vi "02Manejo_panel 568.vi"(0 "Config Equipos":T2(array[cluster]) {"Ref PD" max=10000 step=1; "Med Princ" items=["1", "2", "3", "4", "5", "6", "7", "8", "9", "10", "11", "12", "13", "14", "15", "16", "17", "18", "19", "20", "21", "22", "23", "24", "25", "26", "27", "28", "29", "30", "31", "32"]}, 2 "Med EQ 568":T1, 3 "Nº equipo":i32, 4 "Paneles in":T4(array[cluster]) {"Nº" min=1.0 max=60.0 step=1.0 format="%#2.1f"; "Ultima recepción" format="%<%d/%m - %X>T"; "Med\nPpal" format="%_4g"}) -> (5 "Paneles out":T3(array[cluster]) {"Numeric" min=1.0 max=60.0 step=1.0 format="%#2.1f"; "Ultima recepción" format="%<%d/%m - %X>T"; "Med\nPpal" format="%_4g"})   [LabVIEW 2010]
panel:
  in  "Flags recep":bool[](array[boolean])
  out "T. error":timestamp[](array[timestamp])
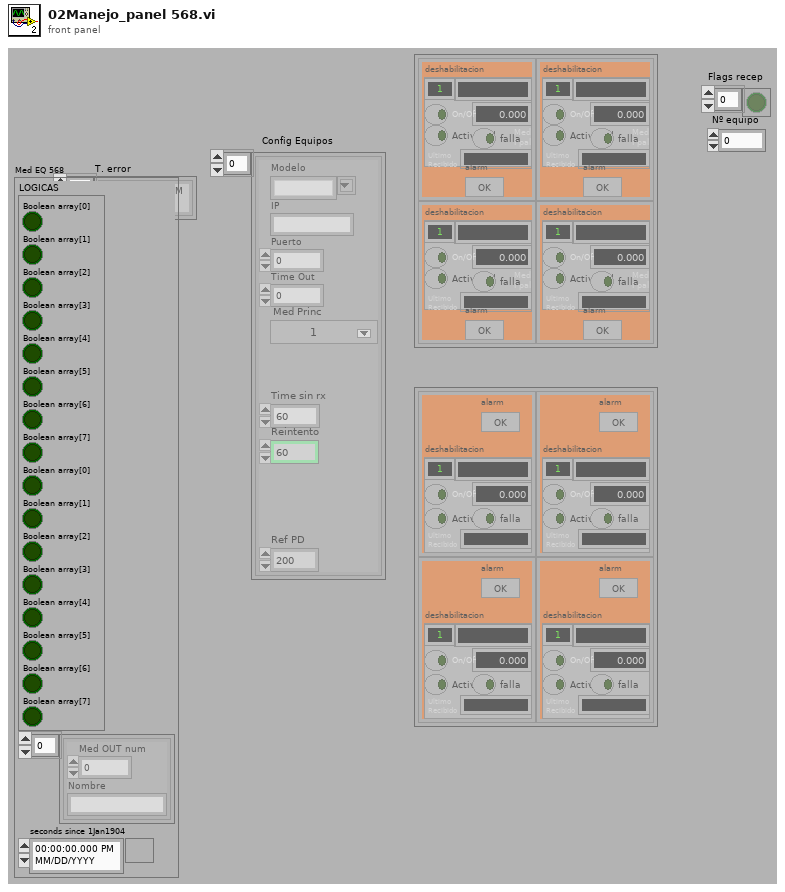
[diagram p1: front panel]
types:
  T1 = cluster{"LOGICAS":cluster{"Boolean array[0]":bool, "Boolean array[1]":bool, "Boolean array[2]":bool, "Boolean array[3]":bool, "Boolean array[4]":bool, "Boolean array[5]":bool, "Boolean array[6]":bool, "Boolean array[7]":bool, "Boolean array[0]":bool, "Boolean array[1]":bool, "Boolean array[2]":bool, "Boolean array[3]":bool, "Boolean array[4]":bool, "Boolean array[5]":bool, "Boolean array[6]":bool, "Boolean array[7]":bool}, cluster{"Med OUT num":dbl, "Nombre":string}[], "seconds since 1Jan1904":timestamp}
  T2 = cluster{"Modelo":string, "IP":string, "Puerto":u16, "Time Out":u16, "Med Princ":u16, "Time sin rx":u16, "Reintento":u16, "Ref PD":u16}[]
  T3 = cluster{"Nombre":string, "Med\nPpal":dbl, "On/Off":bool, "Ultima recepción":timestamp, "Numeric":dbl, "deshabilitacion":bool, "Actividad":bool, "falla":bool, "alarm":bool}[][]
  T4 = cluster{"Nombre":string, "Med\nPpal":dbl, "On/Off":bool, "Ultima recepción":timestamp, "Nº":dbl, "deshabilitacion":bool, "Actividad":bool, "falla":bool, "alarm":bool}[][]
  T5 = cluster{"Boolean array[0]":bool, "Boolean array[1]":bool, "Boolean array[2]":bool, "Boolean array[3]":bool, "Boolean array[4]":bool, "Boolean array[5]":bool, "Boolean array[6]":bool, "Boolean array[7]":bool, "Boolean array[0]":bool, "Boolean array[1]":bool, "Boolean array[2]":bool, "Boolean array[3]":bool, "Boolean array[4]":bool, "Boolean array[5]":bool, "Boolean array[6]":bool, "Boolean array[7]":bool}
  T6 = cluster{"Modelo":string, "IP":string, "Puerto":u16, "Time Out":u16, "Med Princ":u16, "Time sin rx":u16, "Reintento":u16, "Ref PD":u16}
  T7 = cluster{"Nombre":string, "Med\nPpal":dbl, "On/Off":bool, "Ultima recepción":timestamp, "Nº":dbl, "deshabilitacion":bool, "Actividad":bool, "falla":bool, "alarm":bool}
  T8 = cluster{"Nombre":string, "Med OUT num":dbl, "On/Off":bool, "Ultima recepción":timestamp, "Nº":dbl, "deshabilitacion":bool, bool, bool, bool}
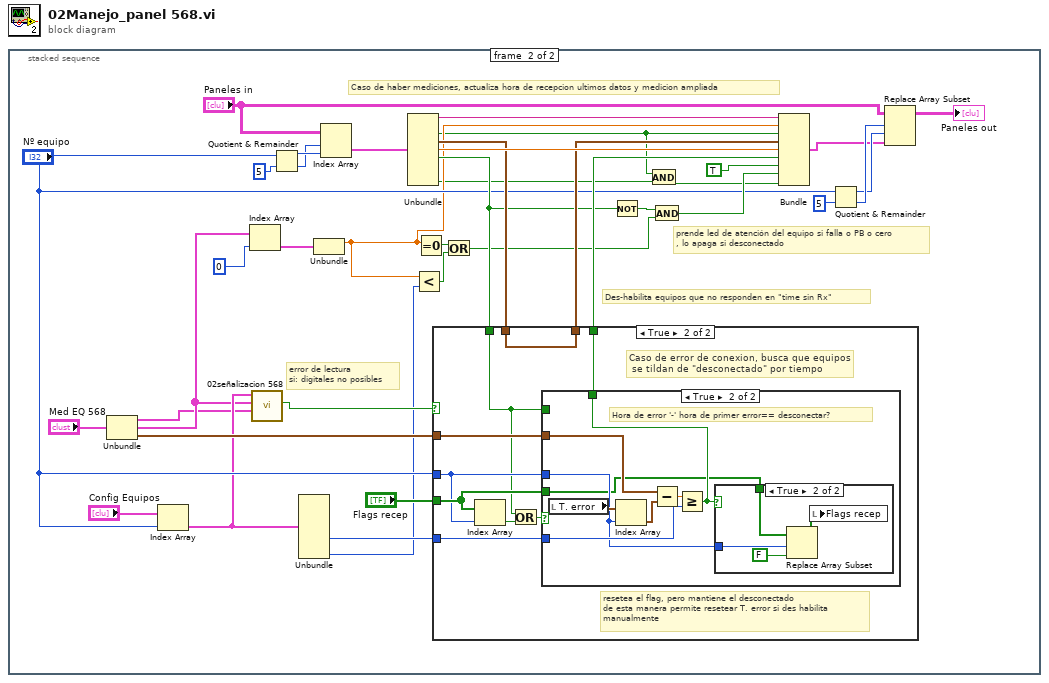
[diagram p0: block diagram]
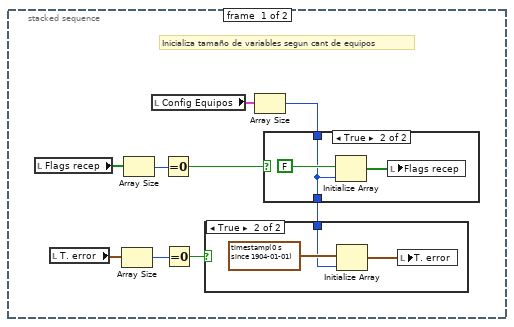
[diagram p2: hidden frame]
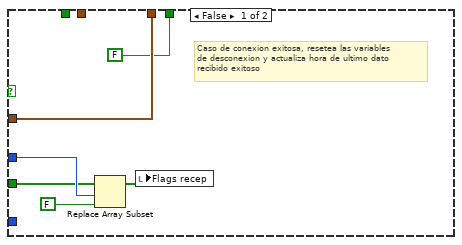
[diagram p5: hidden frame]
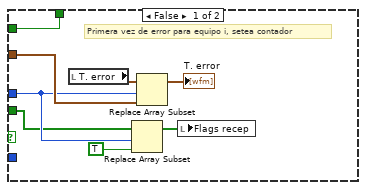
[diagram p6: hidden frame]
diagram:
  n1 = stacked-sequence {
    frame #0 {
      # "Inicializa tamaño de variables segun cant de equipos"
      n2 = local read "Flags recep"() -> (w9:bool[])
      n3 = local read "T. error"() -> (w8:timestamp[])
      n4 = Array Size(array=w8) -> (size(s)=w4:i32)
      n5 = Array Size(array=w9) -> (size(s)=w7:i32)
      n6 = local read "Config Equipos"() -> (w3:T2)
      n7 = Equal To 0?(x=w7) -> (x = 0?=w6:bool)
      n8 = Equal To 0?(x=w4) -> (x = 0?=w5:bool)
      n9 = Array Size(array=w3) -> (size(s)=w2:i32)
      n10 = case shown="True" w6 {
        tunnel: w2 -> [w13 w14]
        tunnel: [w13 w14] -> w1
        frame False {
        }
        frame True {
          n11 = Initialize Array(FALSE, w14) -> (w16:bool[])
          n12 = local write "Flags recep"(w16) -> ()
        }
      }
      n13 = case shown="True" w5 {
        tunnel: w1 -> [_ w10]
        frame False {
        }
        frame True {
          n14 = Initialize Array(timestamp(0 s since 1904-01-01), w10) -> (w12:timestamp[])
          n15 = local write "T. error"(w12) -> ()
        }
      }
    }
    frame #1 {
      # "error de lectura\nsi: digitales no posibles"
      # "prende led de atención del equipo si falla o PB o cero\n, lo apaga si desconectado"
      # "Des-habilita equipos que no responden en \"time sin Rx\""
      # "Caso de haber mediciones, actualiza hora de recepcion ultimos datos y medicion ampliada"
      n16 = Unbundle("Med EQ 568") -> ("LOGICAS"=w26:T5, w27:cluster{"Med OUT num":dbl, "Nombre":string}[], "seconds since 1Jan1904"=w47:timestamp)
      n17 = Index Array(array="Config Equipos", index="Nº equipo") -> (element=w28:T6)
      n18 = Index Array(array=w27, index=0) -> (element=w30:cluster{"Med OUT num":dbl, "Nombre":string})
      n19 = call "02señalizacion 568.vi"("LOGICAS"=w26, "ANALOGICAS"=w27, "Config Equipo"=w28) -> ("Error Logico"=w29:bool)  [unwired: 3 in, 1 out]
      n20 = Quotient & Remainder(x="Nº equipo", y=5) -> (x-y*floor(x/y)=w36:i32, floor(x/y)=w35:i32)
      n21 = Unbundle(w28) -> ("Time sin rx"=w48:u16, "Ref PD"=w24:u16)  [unwired: 6 out]
      n22 = Unbundle(w30) -> ("Med OUT num"=w25:dbl)  [unwired: 1 out]
      n23 = Index Array(array="Paneles in", index (row)=w35, index (col)=w36) -> (element=w34:T7)
      n24 = Unbundle(w34) -> ("Nombre"=w54:string, "On/Off"=w18:bool, "Ultima recepción"=w52:timestamp, "Nº"=w55:dbl, "deshabilitacion"=w46:bool, "alarm"=w19:bool)  [unwired: 3 out]
      n25 = Less?(x=w25, y=w24) -> (x < y?=w22:bool)
      n26 = Equal To 0?(x=w25) -> (x = 0?=w23:bool)
      n27 = case shown="True" w29 {
        tunnel: w47 -> [w61 w69]
        tunnel: [w61 w70] -> w53
        tunnel: w52 -> [_ w70]
        tunnel: w48 -> [_ w68]
        tunnel: "Nº equipo" -> [w58 w66]
        tunnel: "Flags recep" -> [w57 w67]
        tunnel: w46 -> [_ w62]
        tunnel: [FALSE ("new element/subarray") w64] -> w50
        frame False {
          # "Caso de conexion exitosa, resetea las variables\nde desconexion y actualiza hora de ultimo dato\nrecibido exitoso"
          n28 = Replace Array Subset(array=w57, new element=FALSE ("new element/subarray"), index=w58) -> (w60:bool[])
          n29 = local write "Flags recep"(w60) -> ()
        }
        frame True {
          # "resetea el flag, pero mantiene el desconectado\nde esta manera permite resetear T. error si des habilita\nmanualmente"
          # "Caso de error de conexion, busca que equipos\n se tildan de \"desconectado\" por tiempo"
          n30 = Index Array(array=w67, index=w66) -> (element=w63:bool)
          n31 = Or(x=w62, y=w63) -> (x .or. y?=w65:bool)
          n32 = case shown="True" w65 {
            tunnel: w69 -> [w74 w86]
            tunnel: w68 -> [_ w82]
            tunnel: w66 -> [w73 w81]
            tunnel: w67 -> [w72 w79]
            tunnel: w62 -> [w71 _]
            tunnel: [w71 w80] -> w64
            frame False {
              # "Primera vez de error para equipo i, setea contador"
              n33 = local read "T. error"() -> (w78:timestamp[])
              n34 = Replace Array Subset(array=w72, new element=TRUE ("new element/subarray"), index=w73) -> (w76:bool[])
              n35 = Replace Array Subset(array=w78, new element=w74, index=w73) -> (→"T. error":timestamp[])
              n36 = local write "Flags recep"(w76) -> ()
            }
            frame True {
              # "Hora de error '-' hora de primer error== desconectar?"
              n37 = local read "T. error"() -> (w85:timestamp[])
              n38 = Index Array(array=w85, index=w81) -> (element=w84:timestamp)
              n39 = Subtract(x=w86, y=w84) -> (x-y=w83:dbl)
              n40 = Greater Or Equal?(x=w83, y=w82) -> (x >= y?=w80:bool)
              n41 = case shown="True" w80 {
                tunnel: w81 -> [_ w89]
                tunnel: w79 -> [_ w87]
                frame False {
                }
                frame True {
                  n42 = Replace Array Subset(array=w87, new element=FALSE ("new element/subarray"), index=w89) -> (w90:bool[])
                  n43 = local write "Flags recep"(w90) -> ()
                }
              }
            }
          }
        }
      }
      n44 = Or(x=w23, y=w22) -> (x .or. y?=w21:bool)
      n45 = Not(x=w46) -> (.not. x?=w44:bool)
      n46 = And(x=w18, y=w19) -> (x .and. y?=w20:bool)
      n47 = And(x=w44, y=w21) -> (x .and. y?=w45:bool)
      n48 = Bundle("Nombre"=w54, "Med OUT num"=w25, "On/Off"=w18, "Ultima recepción"=w53, "Nº"=w55, "deshabilitacion"=w50, TRUE, w45, w20) -> (w38:T8)  [unwired: 1 out]
      n49 = Quotient & Remainder(x="Nº equipo", y=5) -> (x-y*floor(x/y)=w41:i32, floor(x/y)=w42:i32)
      n50 = Replace Array Subset(array="Paneles in", new element=w38, index (row)=w42, index (col)=w41) -> (→"Paneles out":T4)
    }
  }
